vi "1_2.vi"() -> ()   [LabVIEW 2020]
uses:
  <vilib>/Math Plots/2D Math Plots/2D Error Bar/2D Error Bar Datatype/2D Error Bar Datatype.lvclass
  <vilib>/Math Plots/2D Math Plots/2D Error Bar/2D Error Bar Datatype/Public/Plot Helper (Percentage).vi
panel:
  in  "Blank Button 7":bool caption="Blank Button"
  in  "Blank Button 6":bool caption="Blank Button"
  in  "Blank Button 5":bool caption="Blank Button"
  in  "Dial 2":u16(knob) caption="Starting Phase" scale=0.0..360.0 scale format="%#.6g"
  in  "Boolean 4":bool
  in  "Boolean 3":bool
  in  "Boolean 2":bool
  in  "Blank Button":bool
  in  "Boolean":bool
  out "XY Graph 2":cluster{"X":dbl, "Y":dbl}[](graph)
  out "Slide":u8(slide) caption="Measurement Progress" scale=0.0..100.0
  in  "Dial":u8(knob) scale=0.0..5.0
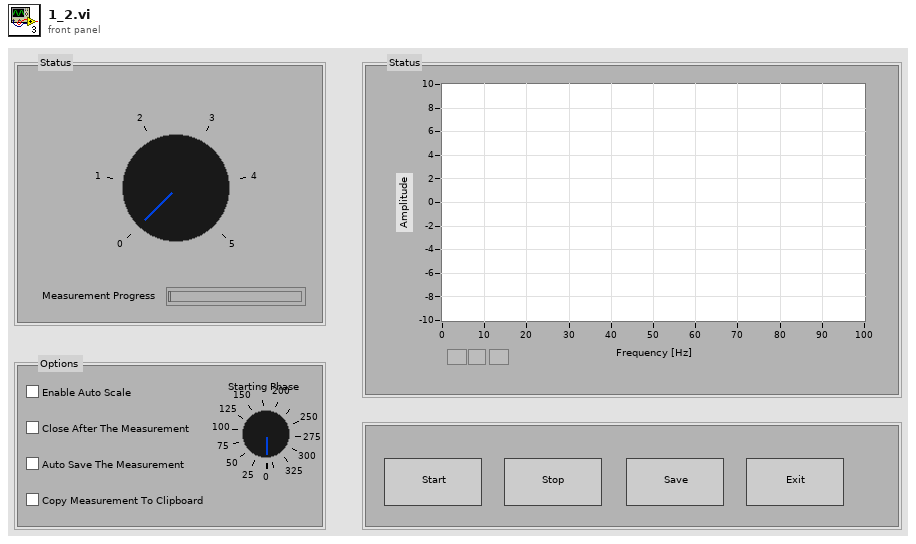
[diagram p1: front panel]
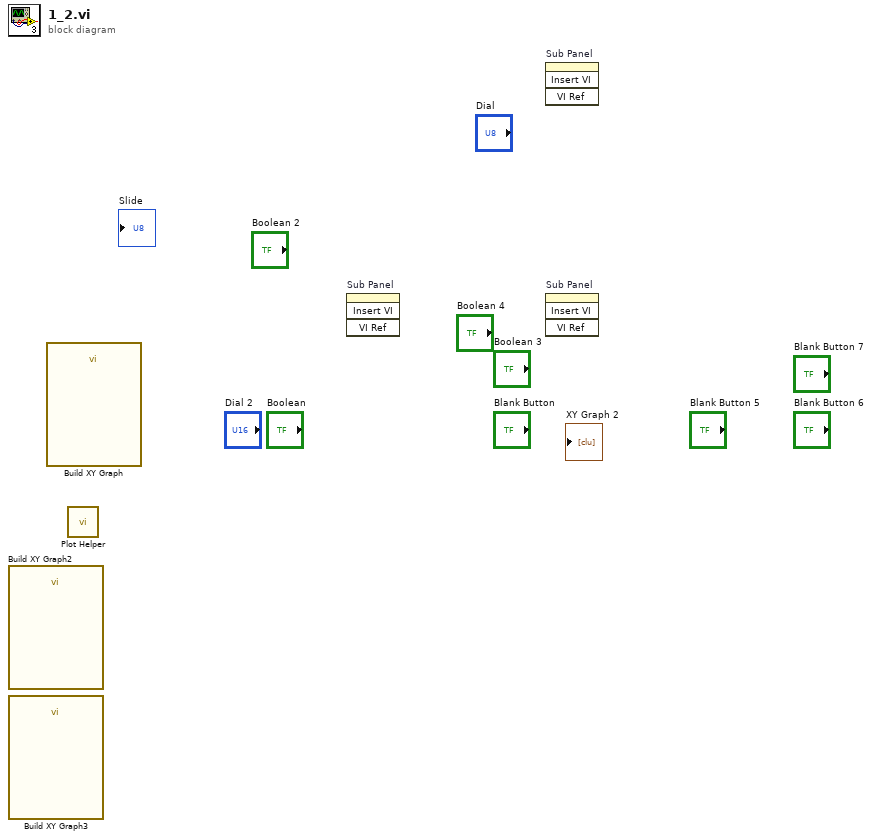
[diagram p0: block diagram]
diagram:
  n1 = call "Build XY Graph2"() -> ()  [unwired: 10 in, 2 out]
  n2 = call "Build XY Graph3"() -> ()  [unwired: 10 in, 2 out]
  n3 = call "Build XY Graph"() -> ()  [unwired: 10 in, 2 out]
  n4 = call-poly <vilib>:"Plot Helper.vi"() -> ()  [unwired: 6 in, 6 out]
  n5 = invoke on="Sub Panel" class="SubPnl" method="Insert VI"() -> ()  [unwired: 4 in, 4 out]
  n6 = invoke on="Sub Panel" class="SubPnl" method="Insert VI"() -> ()  [unwired: 4 in, 4 out]
  n7 = invoke on="Sub Panel" class="SubPnl" method="Insert VI"() -> ()  [unwired: 4 in, 4 out]
